vi "Entry.vi"(8 "error in (no error)":errorcluster, 11 "New State":refnum<class "No Command.lvclass">) -> (0 "error out":errorcluster, 3 "State out":refnum<class "No Command.lvclass">)   [LabVIEW 2014, in "Robot Actor Framework.lvlib" / "Command Processor Actor.lvlib" / "No Command.lvclass"]
doc: "This is an abstract method. Override this method to define the behavior when you enter the state."
uses:
  No Command.lvclass
  Command Processor Actor Class/Command Processor States.ctl
  <vilib>/ActorFramework/Message Enqueuer/Message Priority.ctl
  <vilib>/ActorFramework/Actor/Actor.lvclass/Actor.ctl
  <vilib>/ActorFramework/Message Enqueuer/Message Enqueuer.lvclass/Message Enqueuer.ctl
  <vilib>/ActorFramework/Message Enqueuer/Init from Existing Queue.vi
  <vilib>/ActorFramework/Message Enqueuer/Enqueue.vi
  <vilib>/ActorFramework/Message Priority Queue/Priority Enqueue.vi
  <vilib>/ActorFramework/Message Enqueuer/Message Enqueuer.lvclass
  Command Processor Actor Messages/Go To Starting Command Msg/Go To Starting Command Msg.lvclass
  Command Processor Actor Class/Command Processor Actor.lvclass
  <vilib>/ActorFramework/Actor/Actor.lvclass
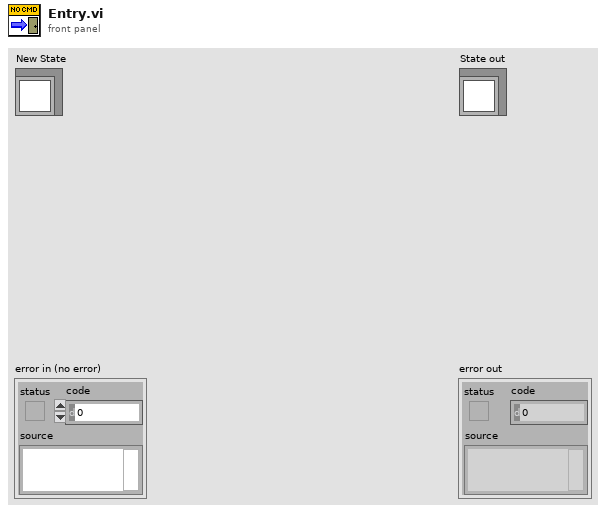
[diagram p1: front panel]
types:
  T1 = typedef "Robot Actor Framework.lvlib/Command Processor Actor.lvlib/Command Processor Actor.lvclass/Command Processor States.ctl" = enum16{"Unknown", "No Command", "Running Command", "Starting Command", "Stopping Command", "Finishing Command"}
  T2 = typedef "Actor Framework.lvlib/Message Enqueuer.lvclass/Message Priority.ctl" = enum16{"Low", "Normal", "High"}
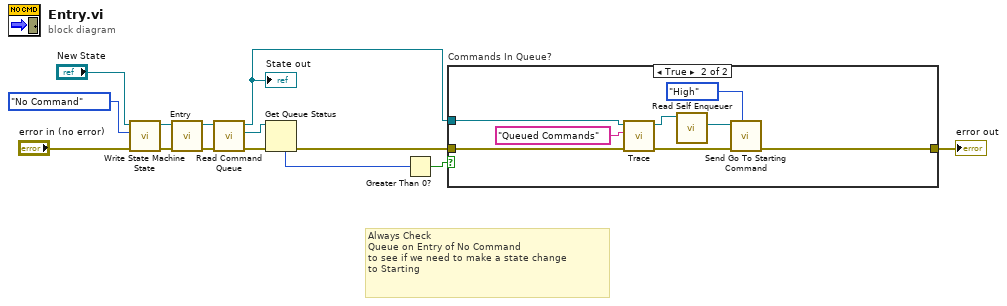
[diagram p0: block diagram]
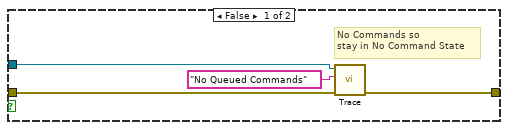
[diagram p2: hidden frame]
diagram:
  # "Always Check\nQueue on Entry of No Command\nto see if we need to make a state change\nto Starting"
  n1 = call-dynamic "Write State Machine State.vi"("error in (no error)"="error in (no error)", "Command Processor State"=Command_Processor_States."No Command", "Command Processor Actor in"="New State") -> ("error out"=w5:errorcluster, "Command Processor Actor out"=w3:refnum<class "No Command.lvclass">)  [unwired: 7 in]
  n2 = call-parent "Entry.vi"("error in (no error)"=w5, "New State"=w3) -> ("error out"=w11:errorcluster, "State out"=w9:refnum<class "No Command.lvclass">)  [unwired: 8 in]
  n3 = call-dynamic "Read Command Queue.vi"("error in (no error)"=w11, "Command Processor Actor in"=w9) -> ("error out"=w10:errorcluster, "Queued Commands"=w14:refnum<queue>, "Command Processor Actor out"=w8:refnum<class "No Command.lvclass">)  [unwired: 7 in]
  "State out" <- w8
  n4 = Get Queue Status(queue=w14, error in (no error)=w10) -> (error out=w2:errorcluster, # elements in queue=w12:i32)  [unwired: 1 in, 6 out]
  n5 = Greater Than 0?(x=w12) -> (x > 0?=w13:bool)
  n6 = case "Commands In Queue?" shown="True" w13 {
    tunnel: w8 -> [w18 w21]
    tunnel: w2 -> [w17 w23]
    tunnel: [w16 w24] -> w1
    frame False {
      # "No Commands so \nstay in No Command State"
      n7 = call-dynamic "Trace.vi"("error in (no error)"=w17, "Command Processor Action"="No Queued Commands", "Command Processor Actor in"=w18) -> ("error out"=w16:errorcluster)  [unwired: 7 in, 1 out]
    }
    frame True {
      n8 = call-dynamic "Trace.vi"("error in (no error)"=w23, "Command Processor Action"="Queued Commands", "Command Processor Actor in"=w21) -> ("error out"=w22:errorcluster, "Command Processor Actor out"=w20:refnum<class "No Command.lvclass">)  [unwired: 7 in]
      n9 = call <vilib>:"Read Self Enqueuer.vi"("Actor"=w20) -> ("Self Enqueuer"=w26:refnum<class "Message Enqueuer.lvclass">)  [unwired: 10 in]
      n10 = call "Send Go To Starting Command.vi"("Message Priority (Normal)"=Message_Priority."High", "error in (no error)"=w22, "Message Enqueuer"=w26) -> ("error out"=w24:errorcluster)  [unwired: 7 in, 1 out]
    }
  }
  "error out" <- w1
